vi "Smart Factory Demo v2.vi"() -> ()   [LabVIEW 2015]
uses:
  <vilib>/Utility/tdmsutil.llb/fileViewerConfigData.ctl
  <vilib>/addons/_XControls/Orbit Plot/SVX Orbit.xctl
panel:
  in  "Boolean":bool
  in  "OK Button 5":bool
  in  "OK Button 4":bool
  in  "stop":bool
  out "LastXScaleFormat":u8
  out "TotalCount":u64
  out "Temp Configuration":T1
  in  "LastTopLeftValue":u64
  out "Resize?":bool
  in  "Help":bool
  out "file path out":path
  in  "Status":string
  in  "Quit":bool
  in  "Settings...":bool
  out "error out":errorcluster
  in  "error in (no error)":errorcluster
  in  "file path":path
  in  "Boolean Text.Text":string
  in  "Color Box 2":u32(colorbox)
  in  "Color Box":u32(colorbox)
  in  "Change Color":bool
  in  "Tab Control":T2(tab)
  out "Boolean 3":bool
  out "Boolean 5":bool
  out "Boolean 2":bool
  out "Waveform Chart 2":dbl(graph)
  out "Waveform Chart":dbl(graph)
  out "Waveform Graph":waveform(dbl)[](graph)
  in  "File contents":string(tree)
  out "Orbit Plot":T3(xcontrol)
  out "Full Spectrum":T4(graph)
  out "Voltage Harmonic Spectra":T5(graph)
  in  "Raw Data":string[][](table)=[["3", "4", "1", "6", "2"], ["33", "26", "12", "100", "23"], ["4", "3", "1", "8", "2"], ["4", "8", "4", "12", "4"], ["2", "3", "1", "9", "3"], ["3", "2", "3", "12", "1"]]
  out "Stacked Bar Plots":dbl[][](graph)
  in  "Stop":bool
  in  "OK Button 3":bool
  in  "OK Button 2":bool
  in  "OK Button":bool
  # "PM-B203\n(Pump B2 #3/4)\n471 days elasped"
  # "dsfsdfofefef"
  # "Smart Factory Demonstration"
  # "Dashboard"
  # "Taipei, Taiwan"
  # "Warning"
  # "Alarm"
  # "Used storage"
  # "Equipment Overview"
  # "BL-A001\n(Blower A0 #1/2)\n471 days elasped"
  # "BL-A002\n(Blower A0 #2/2)\n23 days elasped"
  # "PM-B201\n(Pump B2 #1/4)\n123 days elasped"
  # "PM-B202\n(Pump B2 #2/4)\n71 days elasped"
  # "PM-B204\n(Pump B2 #4/4)\n471 days elasped"
  # "FN-C301\n(Fan C3 #1/5)\n123 days elasped"
  # "FN-C302\n(Fan C3 #2/5)\n123 days elasped"
  # "FN-C303\n(Fan C3 #3/5)\n123 days elasped"
  # "FN-C304\n(Fan C3 #4/5)\n71 days elasped"
  # "FN-C305\n(Fan C3 #5/5)\n471 days elasped"
  # "Overview: Illustrates the use of the waveform graph to display stacked bar plots.\nInstructions:\nRun the VI."
  # "Stacked Bar Waveform Graph.vi"
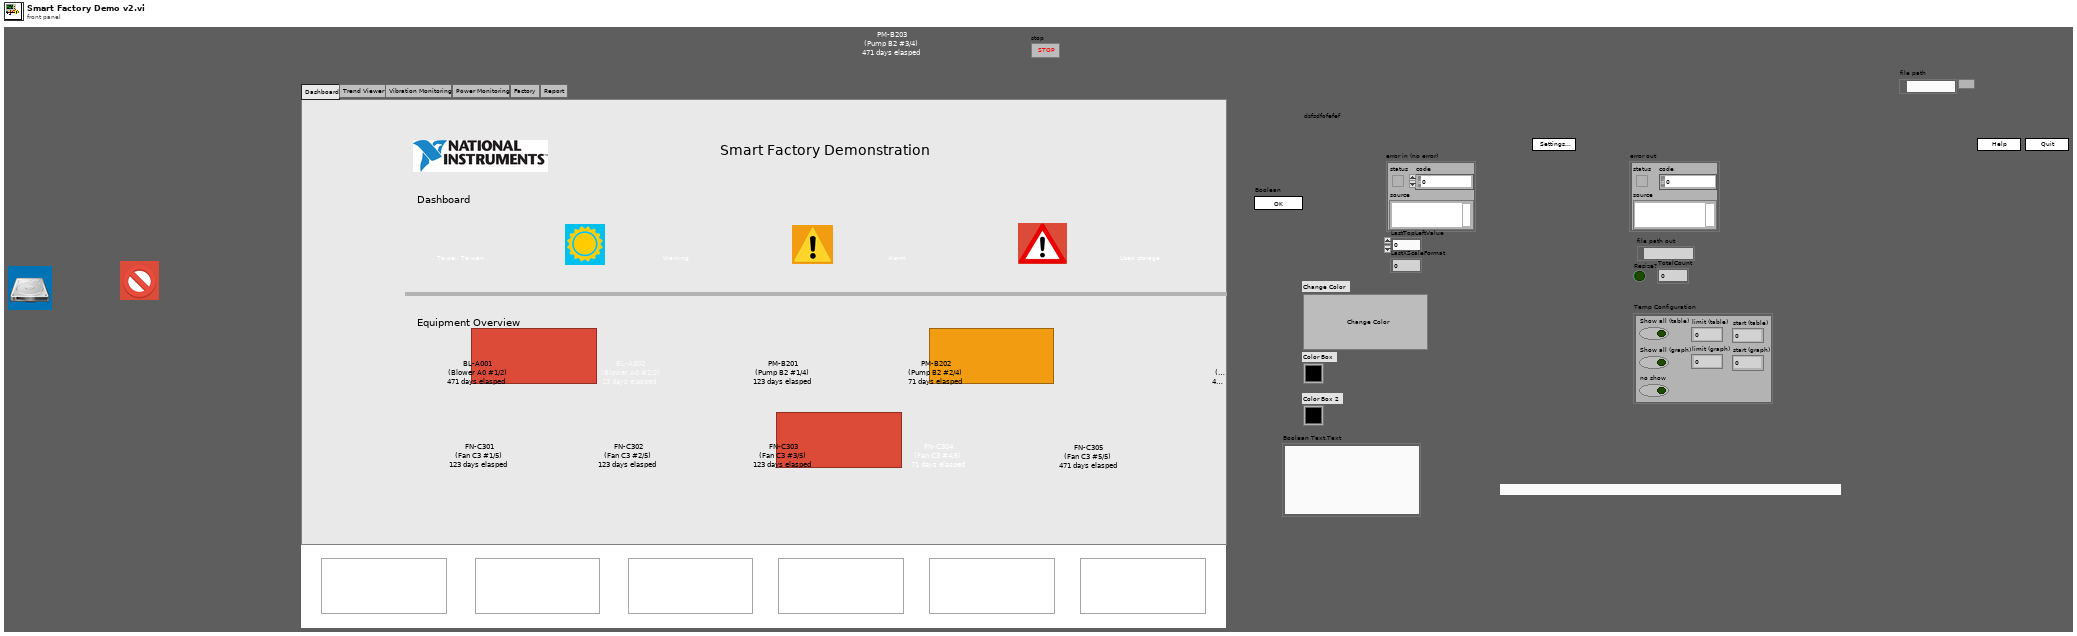
[diagram p1: front panel]
types:
  T1 = typedef "fileViewerConfigData.ctl" = cluster{"Show all (table)":bool, "Show all (graph)":bool, "limit (table)":u64, "limit (graph)":u64, "no show":bool, "start (table)":u64, "start (graph)":u64}
  T2 = enum32{"Dashboard", "Trend Viewer", "Vibration Monitoring", "Power Monitoring", "Factory", "Report"}
  T3 = cluster{"probe x":dbl[], "probe y":dbl[], "reference":dbl[], "plot type":enum16{"Filtered Plot", "Unfiltered Plot"}, "attribute":variant}[][]
  T4 = cluster{"Order 0":dbl, "dOrder":dbl, "magnitude":dbl[]}[]
  T5 = cluster{"order 0":dbl, "delta order":dbl, "complex spectrum":dbl[]}[]
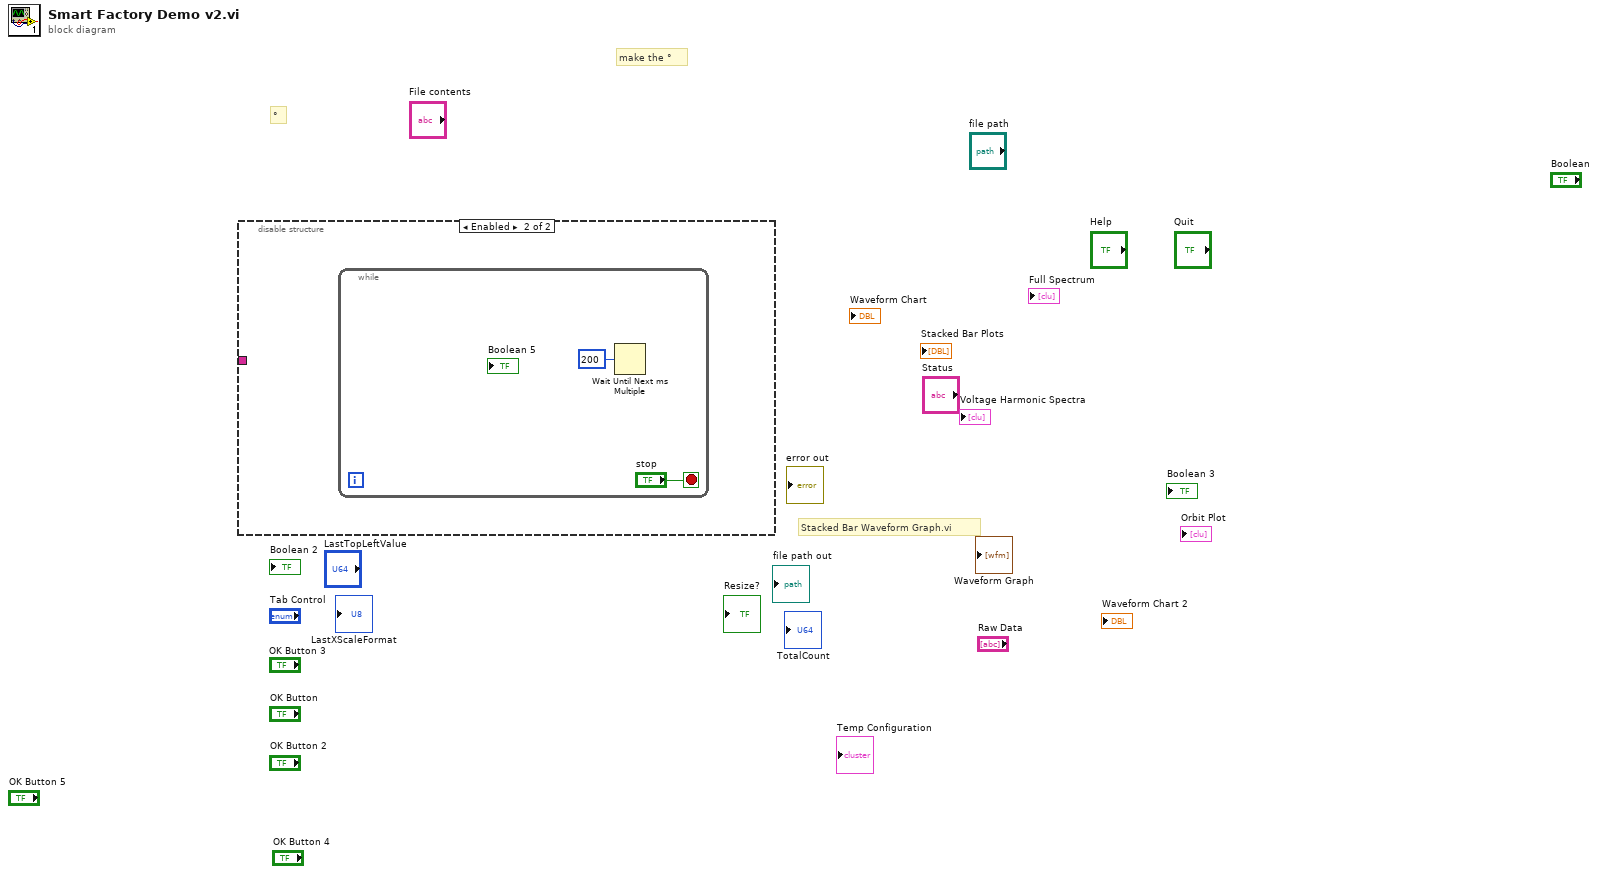
[diagram p0: block diagram]
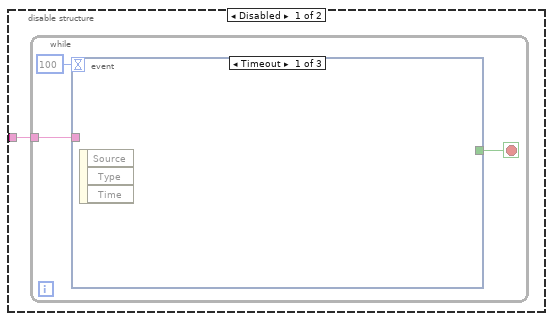
[diagram p2: hidden frame]
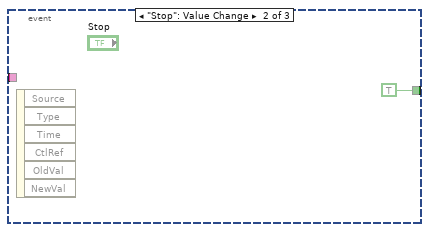
[diagram p3: hidden frame]
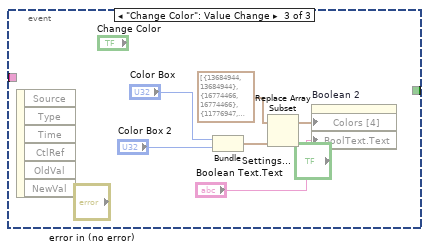
[diagram p4: hidden frame]
diagram:
  # "make the °"
  # "°"
  # "Stacked Bar Waveform Graph.vi"
  n1 = disable-structure shown="Enabled" {
    disable-tunnel: _ -> [w1 _]
    frame Disabled {
      n2 = while {
        tunnel: w1 -> [w2]
        stop <- w4 stop-if-true
        n3 = event shown="[0] Timeout" {
          selector: _ -> [_ _ _]
          dyn-events: _ -> [_ _ _]
          timeout: 100 -> [_ _ _]
          tunnel: [_ TRUE _] -> w4
          tunnel: w2 -> [_ _ _]
          event Timeout {
            n4 = event-data() -> ()  [unwired: 1 in, 3 out]
          }
          event "Stop": Value Change {
            n5 = event-data() -> ()  [unwired: 1 in, 6 out]
          }
          event "Change Color": Value Change {
            n6 = event-data() -> ()  [unwired: 1 in, 6 out]
            n7 = Bundle("Color Box"="Color Box", "Color Box 2"="Color Box 2") -> (w8:cluster{"Color Box":u32, "Color Box 2":u32})  [unwired: 1 in]
            n8 = Replace Array Subset(array=cluster{u32, u32}[] [{13684944, 13684944}, {16774466, 16774466}, {11776947, 39168}, {11776947, 39168}] ("Colors [4]"), new element=w8) -> (w7:cluster{u32, u32}[])  [unwired: 1 in]
            n9 = property on="Boolean 2" class="Bool (strict)"("Colors [4]"=w7, "BoolText.Text"="Boolean Text.Text") -> ()  [unwired: 2 in, 2 out]
          }
        }
      }
    }
    frame Enabled {
      n10 = while {
        stop <- "stop" stop-if-true
        n11 = Wait Until Next ms Multiple(millisecond multiple=u32 200) -> ()  [unwired: 1 out]
      }
    }
  }
